vi "MainComputer.vi"() -> ()   [LabVIEW 2016]
uses:
  Data.ctl
  MainStates.ctl
  <vilib>/Analysis/baseanly.llb/Mean (DBL).vi
  <vilib>/Analysis/NI_AALBase.lvlib
panel:
  in  "IP Address (type in the myRIO IP)":string="172.22.11.2"
  out "error out":errorcluster
  in  "Start Calibration":bool
  in  "Calibration Time (s)":i32=2
  in  "Acquire":bool
  out "myComputer States":T1
  out "Calibrate Data":T2
  out "Waveform Chart":T3(graph)
  in  "stop":bool
  # "Instruction:\n1. Rebuild the distrubution for myRIO (Project windows>myRIO>Build Specification>\"Right Click\" My Source Distribution>Build)\n2. Deploy the Source Distribution (Same location above, Click Deploy)\n3. Run this VI\n4. Click Acquire to obtain the acceleration that detect by the VI in the myRIO (That VI on myRIO is called to run in the \"Start Remote VI\" state in this VI)"
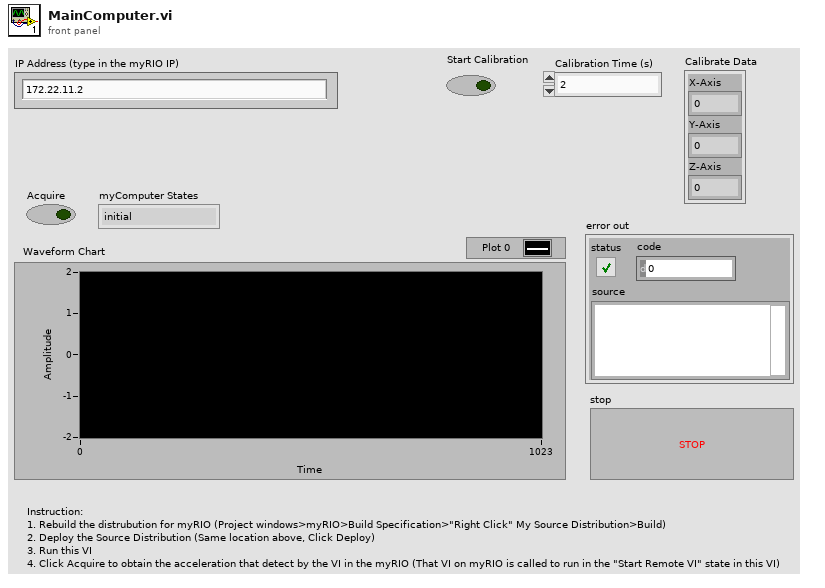
[diagram p1: front panel]
types:
  T1 = typedef "MainStates.ctl" = enum16{"initial", "Start Remote VI", "Calibration", "Wait for input", "Measure", "Stop"}
  T2 = typedef "Data.ctl" = cluster{"X-Axis":dbl, "Y-Axis":dbl, "Z-Axis":dbl}
  T3 = cluster{"X-Axis":dbl, "Y-Axis":dbl, "Z-Axis":dbl}
  T4 = cluster{"application reference":refnum<vi>, "vi reference":refnum<vi>}
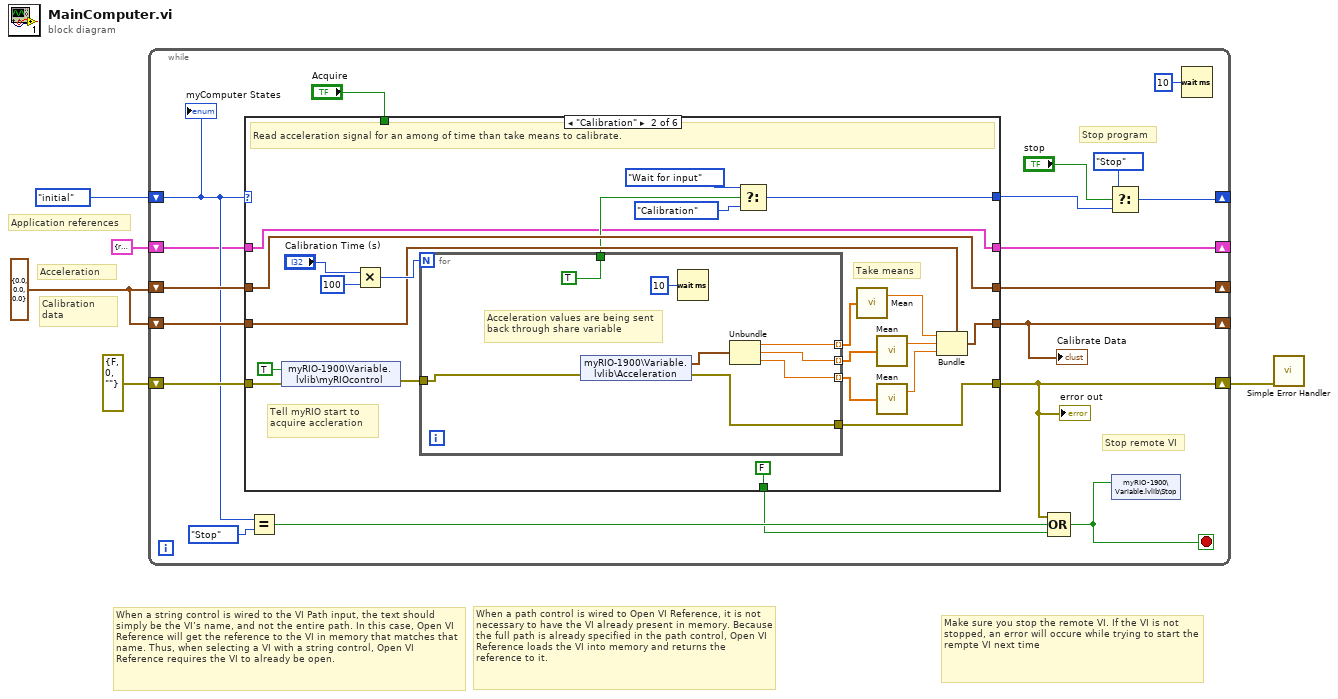
[diagram p0: block diagram]
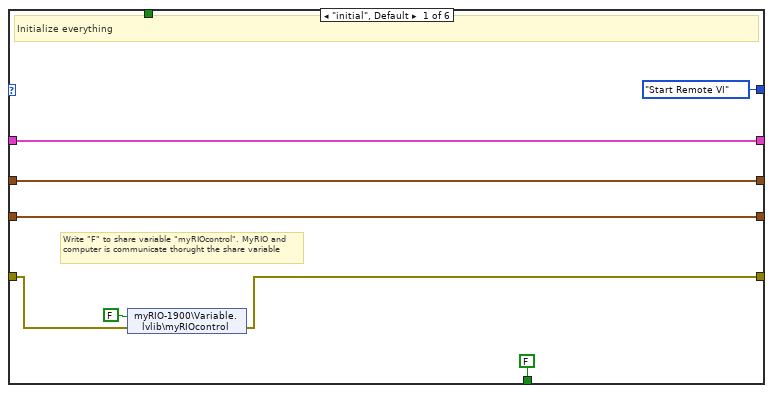
[diagram p2: hidden frame]
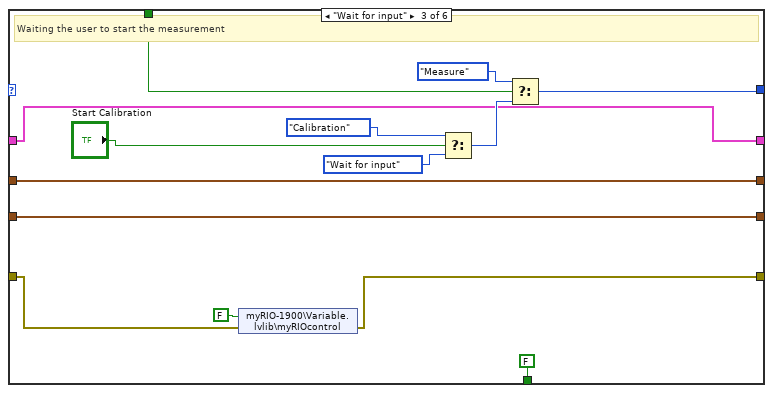
[diagram p3: hidden frame]
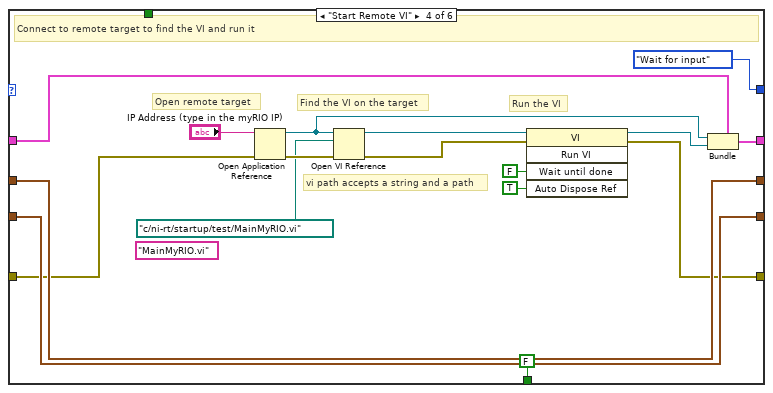
[diagram p4: hidden frame]
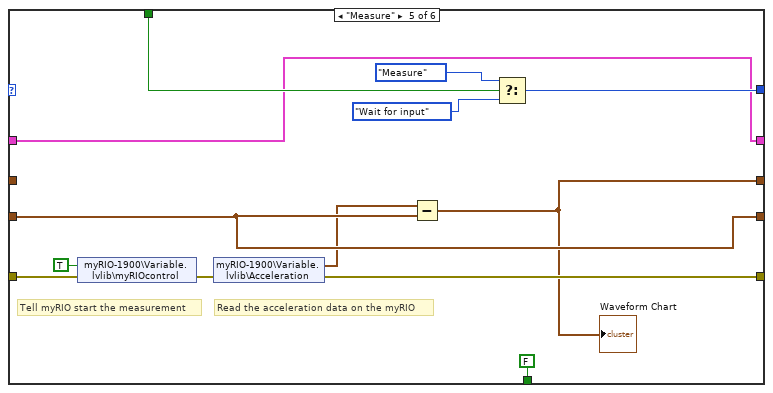
[diagram p5: hidden frame]
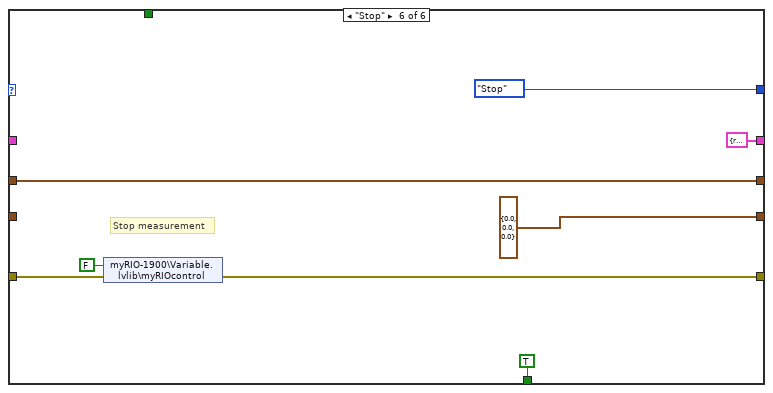
[diagram p6: hidden frame]
diagram:
  w3 = T2 {"X-Axis"=0.0, "Y-Axis"=0.0, "Z-Axis"=0.0} ("Acceleration")
  # "Application references"
  # "Calibration data"
  # "Acceleration"
  # "Make sure you stop the remote VI. If the VI is not stopped, an error will occure while trying to start the rempte VI next time"
  # "When a path control is wired to Open VI Reference, it is not necessary to have the VI already present in memory. Because the full path is already specified in the path control, Open VI Reference loads the VI into memory and returns the reference to it."
  # "When a string control is wired to the VI Path input, the text should simply be the VI’s name, and not the entire path. In this case, Open VI Reference will get the reference to the VI in memory that matches that name. Thus, when selecting a VI with a string control, Open VI Reference requires the VI to already be open."
  n1 = while {
    shift-right: [w21] -> _
    shift-left: MainStates."initial" -> [w14]
    shift-right: [w19] -> _
    shift-left: w3 -> [w20]
    shift-right: [w16] -> w1
    shift-left: errorcluster {"status"=FALSE, "code"=0, "source"=""} ("error constant") -> [w18]
    shift-right: [w10] -> _
    shift-left: w3 -> [w17]
    shift-right: [w8] -> _
    shift-left: T4 {"application reference"=refnum, "vi reference"=refnum} -> [w7]
    stop <- w6 stop-if-true
    # "Stop program"
    # "Stop remote VI"
    n2 = case shown="\"Calibration\"" w14 {
      tunnel: [MainStates."Start Remote VI" w52 w75 MainStates."Wait for input" w101 MainStates."Stop" ("t")] -> w23
      tunnel: w20 -> [w31 w38 w74 w88 _ w114]
      tunnel: [w31 w38 w74 w88 w97 w114] -> w19
      tunnel: w18 -> [w28 w51 w72 w86 w106 w111]
      tunnel: [w25 w36 w71 w84 w103 w108] -> w16
      tunnel: [w29 w39 w73 w87 w102 T2 {"X-Axis"=0.0, "Y-Axis"=0.0, "Z-Axis"=0.0} ("Acceleration")] -> w10
      tunnel: w17 -> [w29 w43 w73 w87 w102 _]
      tunnel: [FALSE FALSE FALSE FALSE FALSE TRUE] -> w12
      tunnel: "Acquire" -> [_ _ w70 _ w98 _]
      tunnel: [w26 w34 w64 w91 w95 T4 {"application reference"=refnum, "vi reference"=refnum}] -> w8
      tunnel: w7 -> [w26 w34 w64 w92 w95 _]
      frame "initial", Default {
        # "Write \"F\" to share variable \"myRIOcontrol\". MyRIO and computer is communicate thorught the share variable"
        # "Initialize everything"
        n3 = shared-variable "myRIO-1900\\Variable.lvlib\\myRIOcontrol"(FALSE ("myRIOcontrol"), error in=w28) -> (error out=w25:errorcluster)
      }
      frame "Calibration" {
        # "Take means"
        # "Tell myRIO start to acquire accleration"
        # "Read acceleration signal for an among of time than take means to calibrate."
        n4 = shared-variable "myRIO-1900\\Variable.lvlib\\myRIOcontrol"(TRUE ("myRIOcontrol"), error in=w51) -> (error out=w50:errorcluster)
        n5 = Multiply(x="Calibration Time (s)", y=100) -> (x*y=w47:i32)
        n6 = for {
          N: w47 -> [_]
          tunnel: w50 -> [w56]
          tunnel: [w60] -> w46 mode=indexing
          tunnel: [w59] -> w45 mode=indexing
          tunnel: [w58] -> w44 mode=indexing
          tunnel: [TRUE ("s")] -> w37
          tunnel: [w55] -> w36
          # "Acceleration values are being sent back through share variable"
          n7 = shared-variable "myRIO-1900\\Variable.lvlib\\Acceleration"(error in=w56) -> (w61:T2, error out=w55:errorcluster)
          n8 = Wait (ms)(milliseconds to wait=u32 10) -> ()  [unwired: 1 out]
          n9 = Unbundle(w61) -> ("X-Axis"=w60:dbl, "Y-Axis"=w59:dbl, "Z-Axis"=w58:dbl)
        }
        n10 = Select(t=MainStates."Wait for input", s=w37, f=MainStates."Calibration") -> (s? t:f=w52:T1)
        n11 = call-poly <vilib>:"Mean.vi"("X"=w46) -> ("mean"=w42:dbl)  [unwired: 1 out]
        n12 = call-poly <vilib>:"Mean.vi"("X"=w45) -> ("mean"=w41:dbl)  [unwired: 1 out]
        n13 = call-poly <vilib>:"Mean.vi"("X"=w44) -> ("mean"=w40:dbl)  [unwired: 1 out]
        n14 = Bundle(cluster=w43, "X-Axis"=w42, "Y-Axis"=w41, "Z-Axis"=w40) -> (w39:T2)
      }
      frame "Wait for input" {
        # "Waiting the user to start the measurement"
        n15 = shared-variable "myRIO-1900\\Variable.lvlib\\myRIOcontrol"(FALSE ("myRIOcontrol"), error in=w72) -> (error out=w71:errorcluster)
        n16 = Select(t=MainStates."Calibration", s="Start Calibration", f=MainStates."Wait for input" ("t")) -> (s? t:f=w66:T1)
        n17 = Select(t=MainStates."Measure", s=w70, f=w66) -> (s? t:f=w75:T1)
      }
      frame "Start Remote VI" {
        (unwired) "MainMyRIO.vi"
        # "Run the VI"
        # "Find the VI on the target"
        # "Open remote target"
        # "vi path accepts a string and a path"
        # "Connect to remote target to find the VI and run it"
        n18 = Open Application Reference(8:w86, 11:"IP Address (type in the myRIO IP)") -> (0:w85:errorcluster, 3:w90:refnum<vi>)  [unwired: 2 in]
        n19 = Open VI Reference(application reference (local)=w90, vi path=path "c:/ni-rt/startup/test/MainMyRIO.vi" ("path"), error in (no error)=w85) -> (vi reference=w79:refnum<vi>, error out=w78:errorcluster)  [unwired: 3 in]
        n20 = invoke class="VI" method="Run VI"(reference=w79, error in=w78, "Wait until done"=FALSE ("Wait Until Done"), "Auto Dispose Ref"=TRUE ("Auto Dispose Reference")) -> (reference out=w89:refnum<vi>, error out=w84:errorcluster)  [unwired: 1 in, 3 out]
        n21 = Bundle(cluster=w92, "application reference"=w90, "vi reference"=w89) -> (w91:T4)
      }
      frame "Measure" {
        # "Read the acceleration data on the myRIO"
        # "Tell myRIO start the measurement"
        n22 = shared-variable "myRIO-1900\\Variable.lvlib\\myRIOcontrol"(TRUE ("myRIOcontrol"), error in=w106) -> (error out=w104:errorcluster)
        n23 = shared-variable "myRIO-1900\\Variable.lvlib\\Acceleration"(error in=w104) -> (w96:T2, error out=w103:errorcluster)
        n24 = Subtract(x=w96, y=w102) -> (x-y=w97:T2)
        "Waveform Chart" <- w97
        n25 = Select(t=MainStates."Measure", s=w98, f=MainStates."Wait for input" ("t")) -> (s? t:f=w101:T1)
      }
      frame "Stop" {
        # "Stop measurement"
        n26 = shared-variable "myRIO-1900\\Variable.lvlib\\myRIOcontrol"(FALSE ("myRIOcontrol"), error in=w111) -> (error out=w108:errorcluster)
      }
    }
    "Calibrate Data" <- w10
    "error out" <- w16
    n27 = Equal?(x=w14, y=MainStates."Stop" ("t")) -> (x = y?=w13:bool)
    n28 = Compound Arithmetic op=OR(w16, w13, w12) -> (w6:bool)
    n29 = Select(t=MainStates."Stop", s="stop", f=w23) -> (s? t:f=w21:T1)
    n30 = shared-variable "myRIO-1900\\Variable.lvlib\\Stop"(w6) -> ()  [unwired: 1 in, 1 out]
    n31 = Wait (ms)(milliseconds to wait=u32 10) -> ()  [unwired: 1 out]
    "myComputer States" <- w14
  }
  n32 = call <vilib>:"Simple Error Handler.vi"("error in (no error)"=w1) -> ()  [unwired: 4 in, 5 out]
